vi "Rectangel RectangleOverlap.vi"(1 "bounds1":T2 {"height" format="%.2f"; "width" format="%.2f"; "y" format="%.2f"; "x" format="%.2f"}, 2 "bounds2":T2 {"height" format="%.2f"; "width" format="%.2f"; "y" format="%.2f"; "x" format="%.2f"}, 5 "error in (no error)":errorcluster, 6 "Bound1HasToBeInsideBound2(False)":bool) -> (15 "overlap":bool, 16 "translate1ToNotOverlap":T1 {"y" format="%.2f"; "x" format="%.2f"}, 19 "error out":errorcluster)   [LabVIEW 2016]
doc: "contains"
uses:
  <resource>/Framework/Providers/Open_GDS/UML/General/Rectangle/Rectangle Rectangle2D.ctl
  <resource>/Framework/Providers/Open_GDS/UML/General/Point/Point Point2D.ctl
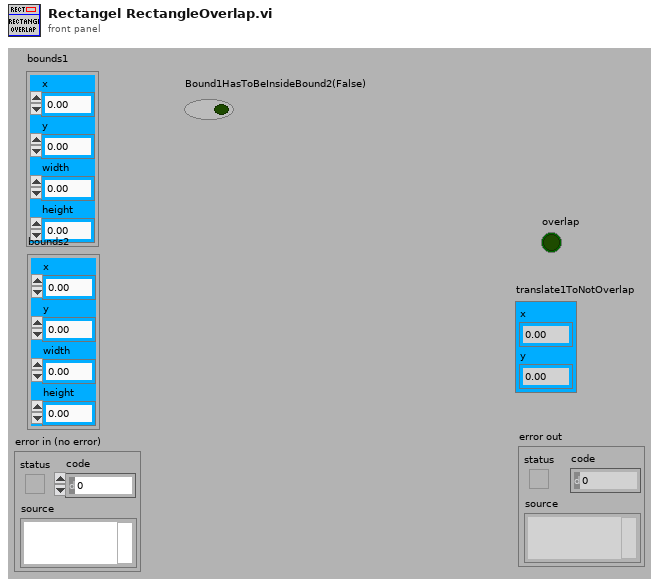
[diagram p1: front panel]
types:
  T1 = typedef "Point Point2D.ctl" = cluster{"x":dbl, "y":dbl}
  T2 = typedef "Rectangle Rectangle2D.ctl" = cluster{"x":dbl, "y":dbl, "width":dbl, "height":dbl}
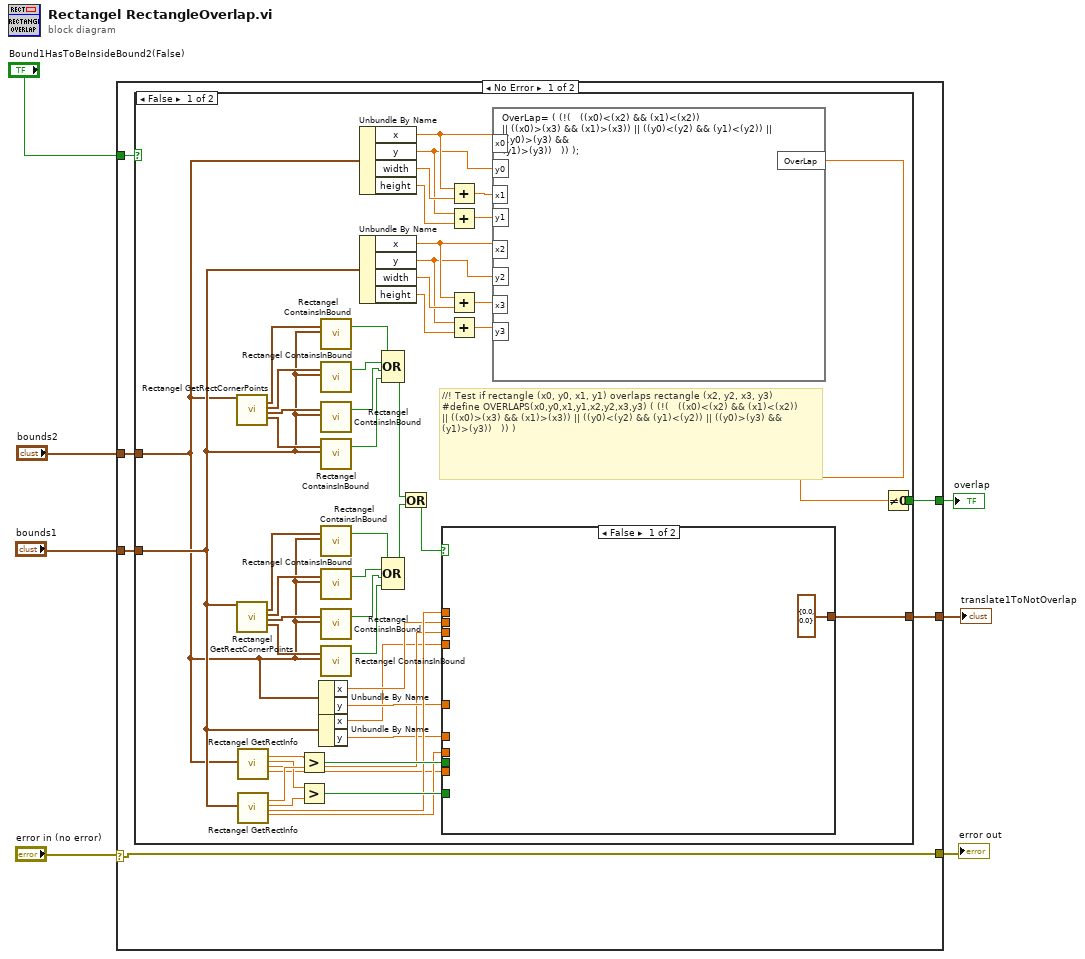
[diagram p0: block diagram]
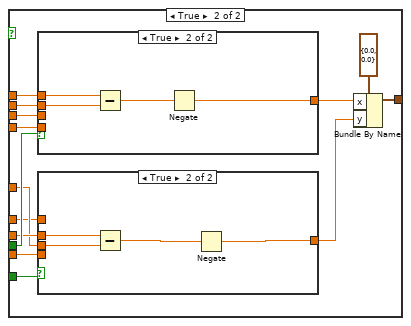
[diagram p2: hidden frame]
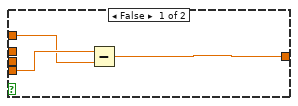
[diagram p3: hidden frame]
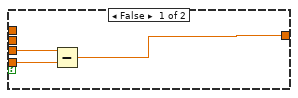
[diagram p4: hidden frame]
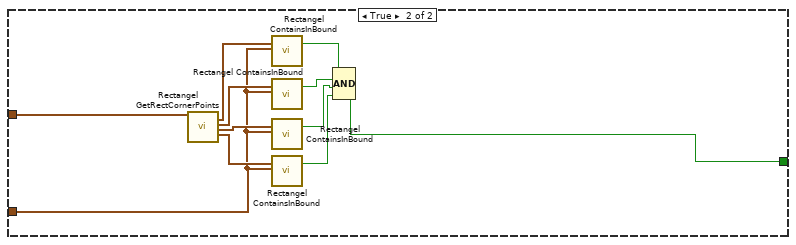
[diagram p5: hidden frame]
diagram:
  n1 = case shown="No Error" "error in (no error)" {
    selector: "error in (no error)" -> [w13 w104]
    tunnel: [w13 w104] -> w7
    tunnel: "bounds1" -> [w11 _]
    tunnel: "bounds2" -> [w10 _]
    tunnel: [w9 _] -> w3
    tunnel: [w12 _] -> w2
    tunnel: "Bound1HasToBeInsideBound2(False)" -> [w8 _]
    frame No Error {
      n2 = case shown="False" w8 {
        tunnel: [w38 _] -> w12
        tunnel: w11 -> [w17 w93]
        tunnel: w10 -> [w16 w94]
        tunnel: [w15 w95] -> w9
        frame False {
          # "//! Test if rectangle (x0, y0, x1, y1) overlaps rectangle (x2, y2, x3, y3)\n#define OVERLAPS(x0,y0,x1,y1,x2,y2,x3,y3) (\t(!(   ((x0)<(x2) && (x1)<(x2))\n|| ((x0)>(x3) && (x1)>(x3)) || ((y0)<(y2) && (y1)<(y2)) || ((y0)>(y3) &&\n(y1)>(y3))   ))\t)"
          n3 = call <resource>:"Rectangel GetRectCornerPoints.vi"("bounds"=w16) -> ("X,Y"=w63:T1, "X+W,Y"=w61:T1, "X,Y+H"=w62:T1, "X+W,Y+H"=w60:T1)  [unwired: 1 in, 14 out]
          n4 = call <resource>:"Rectangel GetRectCornerPoints.vi"("bounds"=w17) -> ("X,Y"=w48:T1, "X+W,Y"=w50:T1, "X,Y+H"=w49:T1, "X+W,Y+H"=w51:T1)  [unwired: 1 in, 14 out]
          n5 = call <resource>:"Rectangel GetRectInfo.vi"("bounds"=w16) -> ("centerX"=w45:dbl, "centerY"=w43:dbl, "maxX"=w33:dbl, "maxY"=w31:dbl)  [unwired: 1 in, 14 out]
          n6 = call <resource>:"Rectangel GetRectInfo.vi"("bounds"=w17) -> ("centerX"=w44:dbl, "centerY"=w42:dbl, "maxX"=w37:dbl, "maxY"=w35:dbl)  [unwired: 1 in, 14 out]
          n7 = Greater?(x=w45, y=w44) -> (0:w41:bool)
          n8 = Greater?(x=w43, y=w42) -> (0:w40:bool)
          n9 = Unbundle By Name(w16) -> ("x"=w36:dbl, "y"=w34:dbl)
          n10 = Unbundle By Name(w17) -> ("x"=w32:dbl, "y"=w30:dbl)
          n11 = call <resource>:"Rectangel ContainsInBound.vi"("point2D"=w63, "bounds"=w17) -> ("contains"=w59:bool)  [unwired: 2 in, 15 out]
          n12 = call <resource>:"Rectangel ContainsInBound.vi"("point2D"=w61, "bounds"=w17) -> ("contains"=w58:bool)  [unwired: 2 in, 15 out]
          n13 = call <resource>:"Rectangel ContainsInBound.vi"("point2D"=w62, "bounds"=w17) -> ("contains"=w57:bool)  [unwired: 2 in, 15 out]
          n14 = call <resource>:"Rectangel ContainsInBound.vi"("point2D"=w60, "bounds"=w17) -> ("contains"=w56:bool)  [unwired: 2 in, 15 out]
          n15 = call <resource>:"Rectangel ContainsInBound.vi"("point2D"=w48, "bounds"=w16) -> ("contains"=w52:bool)  [unwired: 2 in, 15 out]
          n16 = call <resource>:"Rectangel ContainsInBound.vi"("point2D"=w50, "bounds"=w16) -> ("contains"=w53:bool)  [unwired: 2 in, 15 out]
          n17 = call <resource>:"Rectangel ContainsInBound.vi"("point2D"=w49, "bounds"=w16) -> ("contains"=w54:bool)  [unwired: 2 in, 15 out]
          n18 = call <resource>:"Rectangel ContainsInBound.vi"("point2D"=w51, "bounds"=w16) -> ("contains"=w55:bool)  [unwired: 2 in, 15 out]
          n19 = Unbundle By Name(w16) -> ("x"=w29:dbl, "y"=w25:dbl, "width"=w28:dbl, "height"=w24:dbl)
          n20 = Unbundle By Name(w17) -> ("x"=w21:dbl, "y"=w20:dbl, "width"=w22:dbl, "height"=w23:dbl)
          n21 = Compound Arithmetic op=OR(w59, w58, w57, w56) -> (w46:bool)
          n22 = Compound Arithmetic op=OR(w52, w53, w54, w55) -> (w47:bool)
          n23 = Or(x=w46, y=w47) -> (x .or. y?=w39:bool)
          n24 = case shown="False" w39 {
            tunnel: w41 -> [_ w76]
            tunnel: w40 -> [_ w65]
            tunnel: [T1 {"x"=0.0, "y"=0.0} ("translate1ToNotOverlap") w77] -> w38
            tunnel: w37 -> [_ w75]
            tunnel: w36 -> [_ w74]
            tunnel: w35 -> [_ w72]
            tunnel: w34 -> [_ w71]
            tunnel: w33 -> [_ w69]
            tunnel: w32 -> [_ w68]
            tunnel: w31 -> [_ w67]
            tunnel: w30 -> [_ w66]
            frame False {
            }
            frame True {
              n25 = case shown="True" w76 {
                tunnel: w75 -> [_ w92]
                tunnel: w74 -> [_ w91]
                tunnel: [w86 w89] -> w73
                tunnel: w69 -> [w88 _]
                tunnel: w68 -> [w87 _]
                frame False {
                  n26 = Subtract(x=w88, y=w87) -> (x-y=w86:dbl)
                }
                frame True {
                  n27 = Subtract(x=w92, y=w91) -> (x-y=w90:dbl)
                  n28 = Negate(x=w90) -> (-x=w89:dbl)
                }
              }
              n29 = case shown="True" w65 {
                tunnel: w72 -> [_ w85]
                tunnel: w71 -> [_ w84]
                tunnel: [w79 w82] -> w70
                tunnel: w67 -> [w81 _]
                tunnel: w66 -> [w80 _]
                frame False {
                  n30 = Subtract(x=w81, y=w80) -> (x-y=w79:dbl)
                }
                frame True {
                  n31 = Subtract(x=w85, y=w84) -> (x-y=w83:dbl)
                  n32 = Negate(x=w83) -> (-x=w82:dbl)
                }
              }
              n33 = Bundle By Name(cluster=T1 {"x"=0.0, "y"=0.0} ("translate1ToNotOverlap"), "x"=w73, "y"=w70) -> (w77:T1)
            }
          }
          n34 = Add(x=w29, y=w28) -> (x+y=w27:dbl)
          n35 = Add(x=w25, y=w24) -> (x+y=w26:dbl)
          n36 = Add(x=w21, y=w22) -> (x+y=w19:dbl)
          n37 = Add(x=w20, y=w23) -> (x+y=w18:dbl)
          n38 = formula code="OverLap= (\t(!(   ((x0)<(x2) && (x1)<(x2))\n|| ((x0)>(x3) && (x1)>(x3)) || ((y0)<(y2) && (y1)<(y2)) || ((y0)>(y3) &&\n(y1)>(y3))   ))\t);"("x0"=w29, "y0"=w25, "x1"=w27, "y1"=w26, "x2"=w21, "y2"=w20, "x3"=w19, "y3"=w18) -> ("OverLap"=w14:dbl)
          n39 = Not Equal To 0?(x=w14) -> (x != 0?=w15:bool)
        }
        frame True {
          n40 = call <resource>:"Rectangel GetRectCornerPoints.vi"("bounds"=w94) -> ("X,Y"=w103:T1, "X+W,Y"=w101:T1, "X,Y+H"=w102:T1, "X+W,Y+H"=w100:T1)  [unwired: 1 in, 14 out]
          n41 = call <resource>:"Rectangel ContainsInBound.vi"("point2D"=w103, "bounds"=w93) -> ("contains"=w99:bool)  [unwired: 2 in, 15 out]
          n42 = call <resource>:"Rectangel ContainsInBound.vi"("point2D"=w101, "bounds"=w93) -> ("contains"=w98:bool)  [unwired: 2 in, 15 out]
          n43 = call <resource>:"Rectangel ContainsInBound.vi"("point2D"=w102, "bounds"=w93) -> ("contains"=w97:bool)  [unwired: 2 in, 15 out]
          n44 = call <resource>:"Rectangel ContainsInBound.vi"("point2D"=w100, "bounds"=w93) -> ("contains"=w96:bool)  [unwired: 2 in, 15 out]
          n45 = Compound Arithmetic op=AND(w99, w98, w97, w96) -> (w95:bool)
        }
      }
    }
    frame Error {
    }
  }
  "error out" <- w7
  "overlap" <- w3
  "translate1ToNotOverlap" <- w2
